vi "Lift Front Arms (William).vi"(11 "Motor Output":dbl) -> (0 "FrontArmBottom":bool, 3 "FrontArmTop":bool)   [LabVIEW 2014]
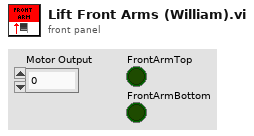
[diagram p1: front panel]
types:
  T1 = typedef "WPI_DigitalInputDevRef.ctl" = cluster{"DevStatus":errorcluster, "DIO Channel":T2, "Controller":T3}
  T2 = typedef "FPGA_DIOChannel.ctl" = enum8{"DIO 0", "DIO 1", "DIO 2", "DIO 3", "DIO 4", "DIO 5", "DIO 6", "DIO 7", "DIO 8", "DIO 9", "DIO MXP 0", "DIO MXP 1", "DIO MXP 2", "DIO MXP 3", "DIO MXP 4", "DIO MXP 5", "DIO MXP 6", "DIO MXP 7", "DIO MXP 8", "DIO MXP 9", "DIO MXP 10", "DIO MXP 11", "DIO MXP 12", "DIO MXP 13", "DIO MXP 14", "DIO MXP 15", "Invalid"}
  T3 = typedef "FPGA_TypedefDigitalModule.ctl" = enum16{"Controller 1"}
  T4 = typedef "WPI_EncoderDevRef.ctl" = cluster{"DevStatus":errorcluster, "EncoderIndex":T5, "CounterIndex":T6, "DistancePerCount":dbl, "Decoding Type":T7}
  T5 = typedef "FPGA_EncoderIdx.ctl" = enum8{"Enc 0", "Enc 1", "Enc 2", "Enc 3", "Enc 4", "Enc 5", "Enc 6", "Enc 7", "Invalid"}
  T6 = typedef "FPGA_CounterCtrSystemIndex.ctl" = enum8{"Ctr 0", "Ctr 1", "Ctr 2", "Ctr 3", "Ctr 4", "Ctr 5", "Ctr 6", "Ctr 7", "Invalid"}
  T7 = typedef "WPI_EncoderType.ctl" = enum16{"1x", "2x", "4x"}
  T8 = typedef "WPI_MotorControlDeviceRef.ctl" = cluster{"DeviceStatus":errorcluster, "Type":T9, "PWM":cluster{"Controller":T3, "PWM Channel":T10, "DeadBand":T11}, "CAN":cluster{"Device Number":u8, "Control Mode":T12, "Semaphore":T13, "Max Vout":dbl, "TalonSRX Control Mode":T14}, "Invert":bool, "TransformRef":T15, "InvTransformRef":T15}
  T9 = typedef "WPI_MotorControlType.ctl" = enum16{"PWM", "CAN", "CANTalonSRX"}
  T10 = typedef "FPGA_DIOPWMChannel.ctl" = enum8{"PWM 0", "PWM 1", "PWM 2", "PWM 3", "PWM 4", "PWM 5", "PWM 6", "PWM 7", "PWM 8", "PWM 9", "PWM MXP 0", "PWM MXP 1", "PWM MXP 2", "PWM MXP 3", "PWM MXP 4", "PWM MXP 5", "PWM MXP 6", "PWM MXP 7", "PWM MXP 8", "PWM MXP 9", "Invalid"}
  T11 = typedef "WPI_PWMDeadband.ctl" = cluster{"Name":string, "maxPositivePwm":i32, "minPositivePwm":i32, "centerPwm":i32, "maxNegativePwm":i32, "minNegativePwm":i32, "angularRange":u16}
  T12 = typedef "WPI_CANJaguar_ControlMode.ctl" = enum8{"Percent VBus", "Current", "Speed", "Position", "Voltage"}
  T13 = typedef "Semaphore RefNum" = refnum<k1>
  T14 = typedef "WPI_CANTalonSRX_APIControlMode.ctl" = enum8{"Percent VBus", "Speed", "Position", "Slave", "Unchanged / Invalid"}
  T15 = typedef "WPI_PWMTransform_ConPane.ctl" = refnum<vi>
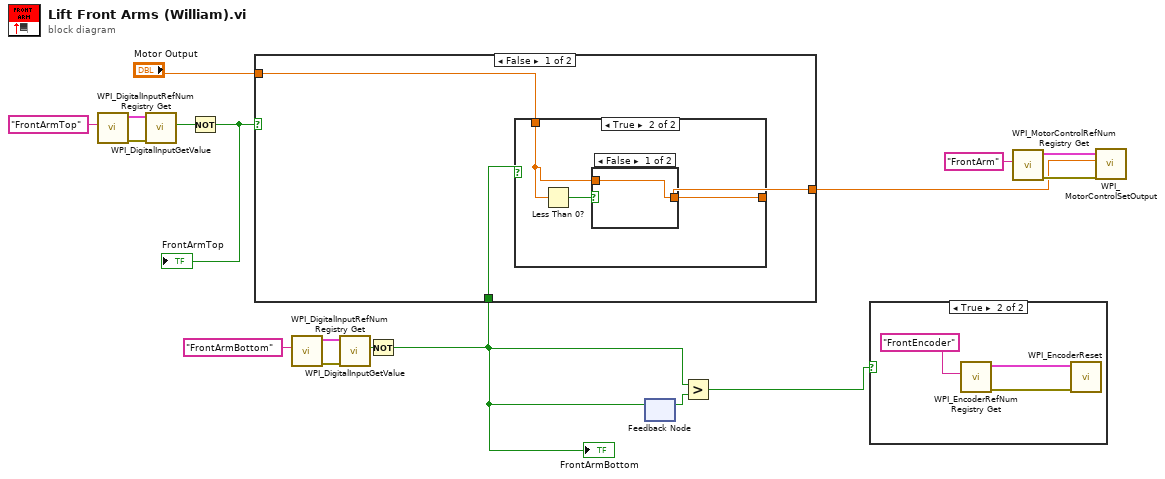
[diagram p0: block diagram]
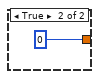
[diagram p4: hidden frame]
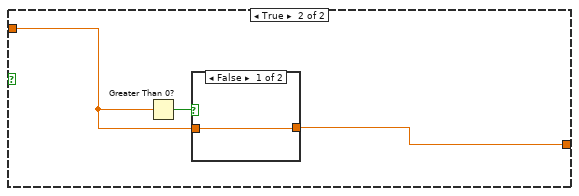
[diagram p5: hidden frame]
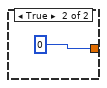
[diagram p6: hidden frame]
diagram:
  n1 = call <vilib>:"WPI_DigitalInputRefNum Registry Get.vi"("refnum name"="FrontArmTop") -> ("error out"=w14:errorcluster, "DigitalInputDevRef"=w13:T1)  [unwired: 9 in]
  n2 = call <vilib>:"WPI_DigitalInputGetValue.vi"("error in (no error)"=w14, "DigitalInputDevRef"=w13) -> ("Value"=w10:bool)  [unwired: 7 in, 2 out]
  n3 = Not(x=w10) -> (.not. x?=w5:bool)
  "FrontArmTop" <- w5
  n4 = call <vilib>:"WPI_DigitalInputRefNum Registry Get.vi"("refnum name"="FrontArmBottom") -> ("error out"=w6:errorcluster, "DigitalInputDevRef"=w7:T1)  [unwired: 9 in]
  n5 = call <vilib>:"WPI_DigitalInputGetValue.vi"("error in (no error)"=w6, "DigitalInputDevRef"=w7) -> ("Value"=w9:bool)  [unwired: 7 in, 2 out]
  n6 = Not(x=w9) -> (.not. x?=w2:bool)
  "FrontArmBottom" <- w2
  n7 = case shown="False" w5 {
    tunnel: "Motor Output" -> [w20 w27]
    tunnel: [w19 w28] -> w4
    tunnel: w2 -> [w18 _]
    frame False {
      n8 = case shown="True" w18 {
        tunnel: w20 -> [w21 w22]
        tunnel: [w21 w23] -> w19
        frame False {
        }
        frame True {
          n9 = Less Than 0?(x=w22) -> (x < 0?=w24:bool)
          n10 = case shown="False" w24 {
            tunnel: [w25 0] -> w23
            tunnel: w22 -> [w25 _]
            frame False {
            }
            frame True {
            }
          }
        }
      }
    }
    frame True {
      n11 = Greater Than 0?(x=w27) -> (x > 0?=w29:bool)
      n12 = case shown="False" w29 {
        tunnel: [w30 0] -> w28
        tunnel: w27 -> [w30 _]
        frame False {
        }
        frame True {
        }
      }
    }
  }
  n13 = feedback #1() -> (w3:bool)  [unwired: 1 in]
  n14 = feedback-in #1(w2) -> ()
  n15 = Greater?(x=w2, y=w3) -> (0:w1:bool)
  n16 = case shown="True" w1 {
    frame False {
    }
    frame True {
      n17 = call <vilib>:"WPI_EncoderRefNum Registry Get.vi"("refnum name"="FrontEncoder") -> ("error out"=w32:errorcluster, "EncoderDevRef"=w34:T4)  [unwired: 9 in]
      n18 = call <vilib>:"WPI_EncoderReset.vi"("error in (no error)"=w32, "EncoderDevRef"=w34) -> ()  [unwired: 8 in, 2 out]
    }
  }
  n19 = call <vilib>:"WPI_MotorControlRefNum Registry Get.vi"("refnum name"="FrontArm") -> ("error out"=w15:errorcluster, "MotorControlDevRef"=w16:T8)  [unwired: 9 in]
  n20 = call <vilib>:"WPI_MotorControlSetOutput.vi"("error in (no error)"=w15, "Output"=w4, "MotorControlDevRef"=w16) -> ()  [unwired: 6 in, 3 out]
